vi "cv_06-01.vi"() -> ()   [LabVIEW 2013]
panel:
  in  "Power":bool
  out "Temperature History":u16(graph)
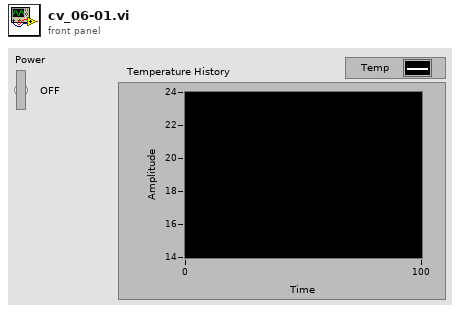
[diagram p1: front panel]
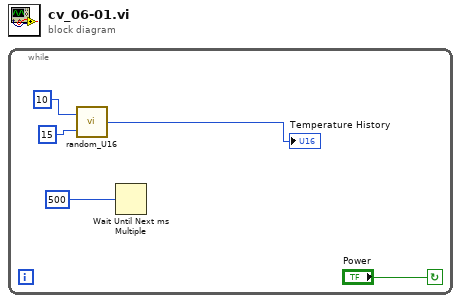
[diagram p0: block diagram]
diagram:
  n1 = while {
    stop <- "Power" continue-if-true
    n2 = call "random_U16.vi"("Offset"=15, "Range"=10) -> ("Out"=→"Temperature History":u16)
    n3 = Wait Until Next ms Multiple(millisecond multiple=500) -> ()  [unwired: 1 out]
  }
